vi "PH_Beckhoff_PPMA-Rods.set Digital Output GUI Elements.vi"(2 "Output GUI Refs":T2, 3 "Digital Outputs":T1, 5 "error in":errorcluster) -> (19 "error out":errorcluster)   [LabVIEW 2014, in "PH_Beckhoff_PPMA-Rods.lvlib"]
doc: "This VI sets the digital Output GUI elements of rod chains and warning lamps."
uses:
  PH_Beckhoff_PPMA-Rods.lvlib
  PH_Beckhoff/PH_Beckhoff.Digital Outputs.ctl
  PH_Beckhoff_PPMA-Rods.Rods Tags.ctl
  PH_Basics/PH_Common/PH_Common.lvlib
  PH_Beckhoff/PH_Beckhoff.lvlib
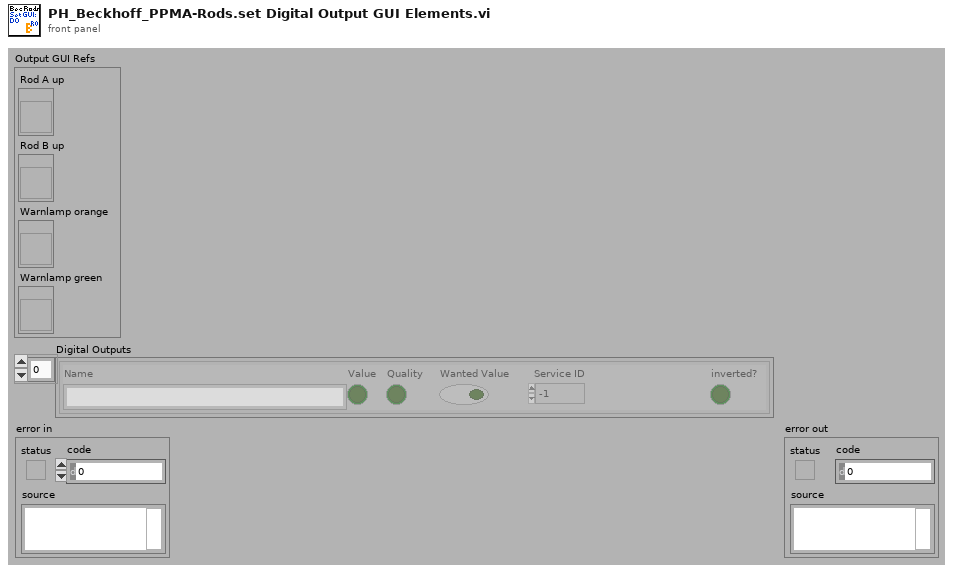
[diagram p1: front panel]
types:
  T1 = typedef "PH_Beckhoff.lvlib/PH_Beckhoff.Digital Outputs.ctl" = cluster{"Name":string, "Value":bool, "Quality":bool, "Wanted Value":bool, "Service ID":i32, "inverted?":bool}[]
  T2 = cluster{"Rod A up":refnum<vi>, "Rod B up":refnum<vi>, "Warnlamp orange":refnum<vi>, "Warnlamp green":refnum<vi>}
  T3 = typedef "PH_Beckhoff_PPMA-Rods.lvlib/PH_Beckhoff_PPMA-Rods.Rods Tags.ctl" = enum16{"Rod-up", "earth-ok", "door-locked-K1", "door-locked-K2", "watervalve-closed", "Rods-Chain-A-up", "Rods-Chain-B-up", "HV-Warnlamp-orange", "HV-Warnlamp-green", "Status-Rods-PU-1", "Status-Rods-PU-2", "Status-Rods-PU-3", "Status-Rods-PU-4", "Status-Rods-PU-5", "Status-Rods-PU-6", "Status-Rods-PU-7", "Status-Rods-PU-8", "Status-Rods-PU-9", "Status-Rods-PU-10", "Status-Rods-FR", "Status-Rods-PILC"}
  T4 = cluster{"Name":string, "Value":bool, "Quality":bool, "Wanted Value":bool, "Service ID":i32, "inverted?":bool}
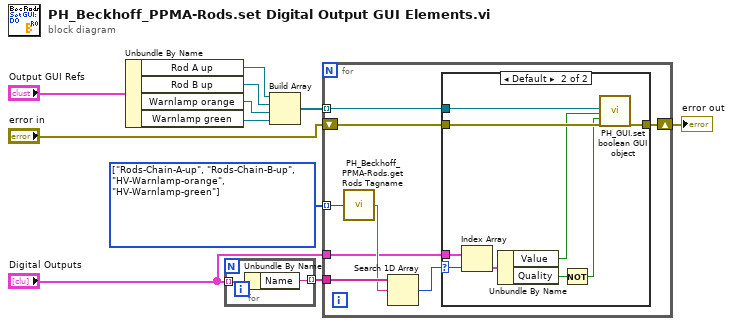
[diagram p0: block diagram]
diagram:
  w8 = T3[] [enum."Rods-Chain-A-up", enum."Rods-Chain-B-up", enum."HV-Warnlamp-orange", enum."HV-Warnlamp-green"] items=["Rod-up", "earth-ok", "door-locked-K1", "door-locked-K2", "watervalve-closed", "Rods-Chain-A-up", "Rods-Chain-B-up", "HV-Warnlamp-orange", "HV-Warnlamp-green", "Status-Rods-PU-1", "Status-Rods-PU-2", "Status-Rods-PU-3", "Status-Rods-PU-4", "Status-Rods-PU-5", "Status-Rods-PU-6", "Status-Rods-PU-7", "Status-Rods-PU-8", "Status-Rods-PU-9", "Status-Rods-PU-10", "Status-Rods-FR", "Status-Rods-PILC"]
  n1 = Unbundle By Name("Output GUI Refs") -> ("Rod A up"=w2:refnum<vi>, "Rod B up"=w3:refnum<vi>, "Warnlamp orange"=w4:refnum<vi>, "Warnlamp green"=w5:refnum<vi>)
  n2 = for {
    tunnel: "Digital Outputs" -> [w13] mode=indexing
    tunnel: [w12] -> w9 mode=indexing
    n3 = Unbundle By Name(w13) -> ("Name"=w12:string)
  }
  n4 = Build Array(w2, w3, w4, w5) -> (w7:refnum<vi>[])
  n5 = for {
    shift-right: [w21] -> w1
    shift-left: "error in" -> [w20]
    tunnel: w7 -> [w19] mode=indexing
    tunnel: w8 -> [w18] mode=indexing
    tunnel: w9 -> [w17]
    tunnel: "Digital Outputs" -> [w15]
    n6 = call "PH_Beckhoff_PPMA-Rods.get Rods Tagname.vi"("Rods Tag"=w18) -> ("Rods Tagname"=w16:string)
    n7 = Search 1D Array(1D array=w17, element=w16) -> (index of element=w14:i32)  [unwired: 1 in]
    n8 = case shown="Default" w14 {
      selector: w14 -> [_ w23]
      tunnel: [w22 w31] -> w21
      tunnel: w20 -> [w22 w30]
      tunnel: w19 -> [_ w29]
      tunnel: w15 -> [_ w28]
      frame -1 {
      }
      frame Default {
        n9 = Index Array(array=w28, index=w23) -> (element=w27:T4)
        n10 = Unbundle By Name(w27) -> ("Value"=w24:bool, "Quality"=w26:bool)
        n11 = Not(x=w26) -> (.not. x?=w25:bool)
        n12 = call "PH_GUI.set boolean GUI object.vi"("Boolean Knob GUI Ref"=w29, "Value"=w24, "Blinking? (false)"=w25, "error in (no error)"=w30) -> ("error out"=w31:errorcluster)  [unwired: 15 in]
      }
    }
  }
  "error out" <- w1
